vi "GetNameOfScaleFile.vi"(8 "Error In":errorcluster) -> (0 "Error Out":errorcluster, 3 "Scale Filename":string)   [LabVIEW 2019]
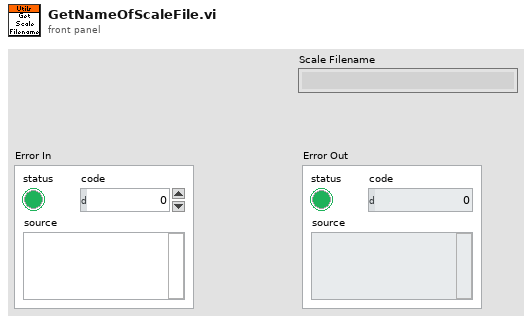
[diagram p1: front panel]
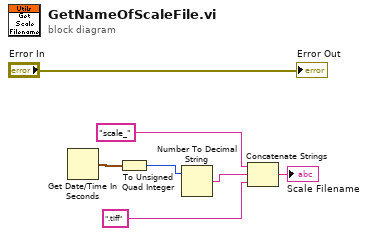
[diagram p0: block diagram]
diagram:
  n1 = Get Date/Time In Seconds() -> (seconds since 1Jan1904=w7:timestamp)
  n2 = To Unsigned Quad Integer(1:w7) -> (0:w6:u64)
  n3 = Number To Decimal String(number=w6) -> (decimal integer string=w4:string)  [unwired: 1 in]
  n4 = Concatenate Strings("scale_", w4, ".tiff" ("string")) -> (→"Scale Filename":string)
  "Error Out" <- "Error In"
